vi "wrap.PullStringArray.vi"(0 "class.GLue in":refnum<class "class.GLue.lvclass">, 7 "Is2d":i32, 11 "error in (no error)":errorcluster, 13 "StringArray in":string[][](array[string])) -> (4 "class.GLue out":refnum<class "class.GLue.lvclass">, 8 "StringArray out":string[][](array[string]), 15 "error out":errorcluster)   [LabVIEW 2014, in "GLue.lvlib" / "class.GLue.lvclass"]
uses:
  class.GLue.lvclass
  class.GLue.lvclass/class.GLue.ctl
  Resources/GLue.dll
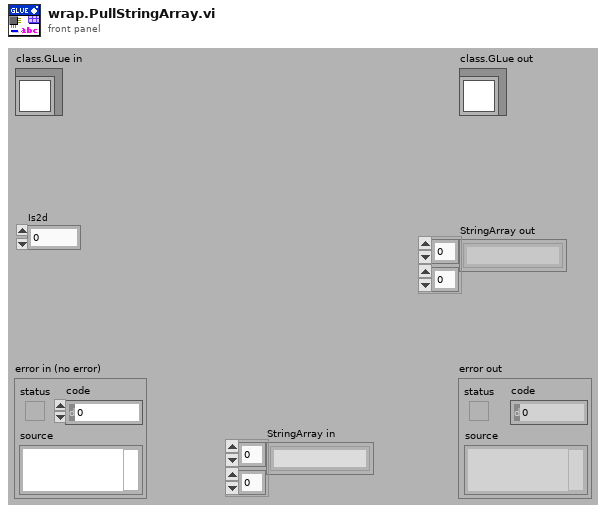
[diagram p1: front panel]
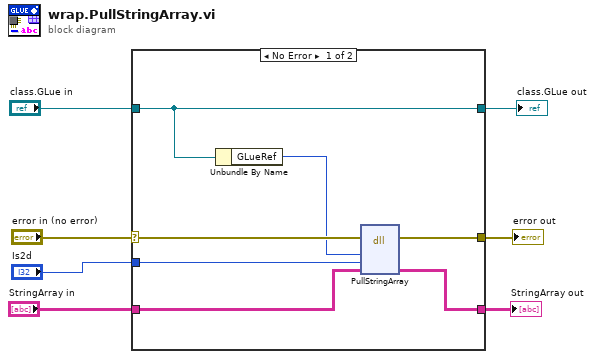
[diagram p0: block diagram]
diagram:
  n1 = case shown="No Error" "error in (no error)" {
    selector: "error in (no error)" -> [w13 w17]
    tunnel: [w12 w17] -> w6
    tunnel: [w14 w16] -> w4
    tunnel: "class.GLue in" -> [w14 w16]
    tunnel: [w10 w15] -> w2
    tunnel: "StringArray in" -> [w9 w15]
    tunnel: "Is2d" -> [w8 _]
    frame No Error {
      n2 = Unbundle By Name(w14) -> ("GLueRef"=w11:i64)
      n3 = dll-call lib="C:/Users/Antonie/Documents/work/glue/trunk/Resources/GLue.dll" fn="PullStringArray"(error in=w13, "MLua"=w11, "Is2d"=w8, "FloatArray"=w9) -> (error out=w12:errorcluster, "FloatArray"=w10:string[][])  [unwired: 5 in, 1 out]
    }
    frame Error {
    }
  }
  "error out" <- w6
  "class.GLue out" <- w4
  "StringArray out" <- w2
